vi "Init CfgFile.vi"(8 "error in (no error)":errorcluster, 11 "LF2R IDE in":refnum<class "LF2R IDE.lvclass">) -> (0 "error out":errorcluster, 3 "LF2R IDE out":refnum<class "LF2R IDE.lvclass">)   [LabVIEW 2018, in "LF2R IDE.lvlib" / "LF2R IDE.lvclass"]
uses:
  LF2R IDE.lvclass
  LF2R IDE.lvclass/LF2R IDE.ctl
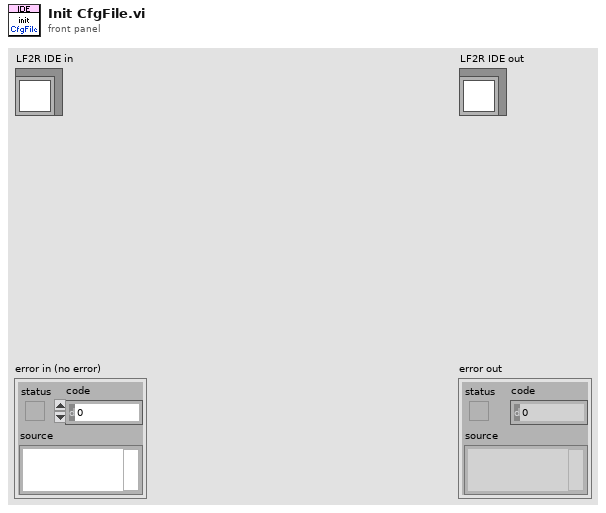
[diagram p1: front panel]
types:
  T1 = typedef "LF2R IDE.lvlib/LF2R IDE.lvclass/Const Configuration.ctl" = cluster{"Language":cluster{"Name":string}, "Path Config":T2, "Image Viewer Config":T3}
  T2 = typedef "LF2R IDE.lvlib/LF2R IDE.lvclass/Const Path Setting.ctl" = cluster{"Data Folder Path":path, "PNG Folder Path":path}
  T3 = typedef "LF2R IDE.lvlib/LF2R IDE.lvclass/Const Image Viewer Setting.ctl" = cluster{"Center Point":cluster{"Size":i32, "Color":u32, "Show?":bool}, "bp Point":cluster{"Size":i32, "Color":u32, "Show?":bool}, "w Point":cluster{"Size":i32, "Color":u32, "Show?":bool}, "b Box":cluster{"Fill Color":u32, "Border Color":u32, "Show?":bool}, "i Box":cluster{"Fill Color":u32, "Border Color":u32, "Show?":bool}, "o Point":cluster{"Size":i32, "Color":u32, "Show?":bool}, "c Point":cluster{"Size":i32, "Color":u32, "Show?":bool}}
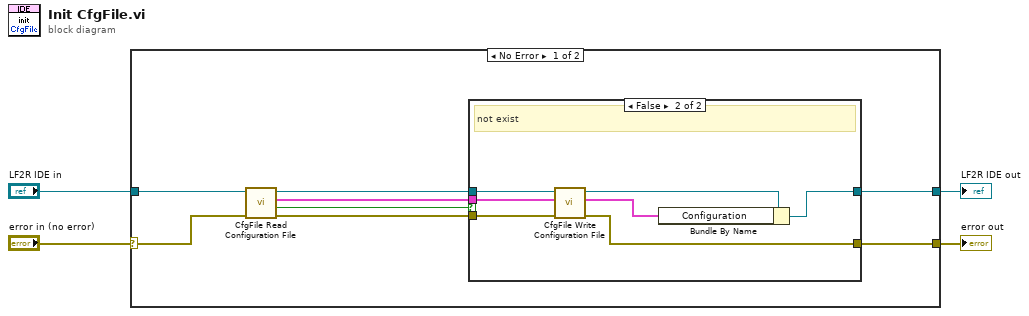
[diagram p0: block diagram]
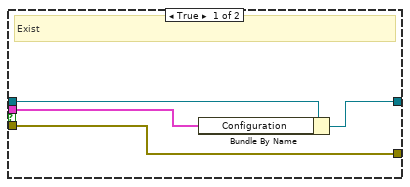
[diagram p2: hidden frame]
diagram:
  n1 = case shown="No Error" "error in (no error)" {
    selector: "error in (no error)" -> [w11 w24]
    tunnel: [w5 w24] -> w3
    tunnel: [w8 w23] -> w1
    tunnel: "LF2R IDE in" -> [w12 w23]
    frame No Error {
      n2 = call "CfgFile Read Configuration File.vi"("error in (no error)"=w11, "LF2R IDE in"=w12) -> ("error out"=w6:errorcluster, "Exist?"=w7:bool, "Config Data"=w9:T1, "LF2R IDE out"=w10:refnum<class "LF2R IDE.lvclass">)  [unwired: 6 in]
      n3 = case shown="False" w7 {
        tunnel: w10 -> [w16 w21]
        tunnel: w9 -> [w15 w18]
        tunnel: [w14 w22] -> w8
        tunnel: w6 -> [w13 w19]
        tunnel: [w13 w17] -> w5
        frame True {
          # "Exist"
          n4 = Bundle By Name(cluster=w16, "Configuration"=w15) -> (w14:refnum<class "LF2R IDE.lvclass">)
        }
        frame False {
          # "not exist"
          n5 = call "CfgFile Write Configuration File.vi"("error in (no error)"=w19, "Configuration"=w18, "LF2R IDE in"=w21) -> ("error out"=w17:errorcluster, "LF2R IDE out"=w20:refnum<class "LF2R IDE.lvclass">)  [unwired: 7 in]
          n6 = Bundle By Name(cluster=w20, "Configuration"=w18) -> (w22:refnum<class "LF2R IDE.lvclass">)
        }
      }
    }
    frame Error {
    }
  }
  "error out" <- w3
  "LF2R IDE out" <- w1
